vi "RSZVB Configure Power Bandwidth Average.vi"(5 "Meas Bandwidth (10.0e3)":dbl=10000.0 format="%^.3e", 6 "Average Factor (10)":i32=10, 7 "Average State (F: Off)":bool, 8 "error in (no error)":errorcluster {"code" format="%.0x"}, 9 "RF State (T: On)":bool=TRUE, 10 "Channel (1)":i32=1, 11 "VISA session":refnum<visa-resource-name>) -> (0 "error out":errorcluster {"code" format="%.0x"}, 3 "dup VISA session":refnum<visa-resource-name>)   [LabVIEW 2011]
doc: "This VI configures the power bandwidth average.\n\nRemote-control command(s):\nDIAGnostic:SERVice:RFPower\n[SENSe<Ch>:]BANDwidth[:RESolution]\n[SENSe<Ch>:]AVERage[:STATe]\n[SENSe<Ch>:]AVERage:COUNt"
panel:
  # "On\nOff"
  # "On\nOff"
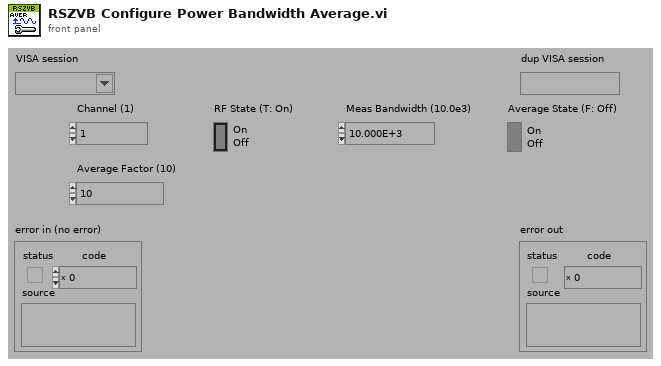
[diagram p1: front panel]
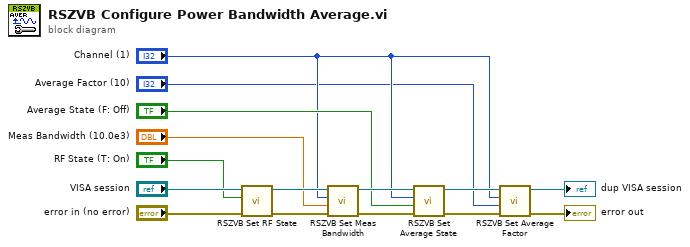
[diagram p0: block diagram]
diagram:
  n1 = call "RSZVB Set RF State.vi"("error in (no error)"="error in (no error)", "RF State (T: On)"="RF State (T: On)", "VISA session"="VISA session") -> ("error out"=w10:errorcluster, "dup VISA session"=w11:refnum<visa-resource-name>)  [unwired: 7 in]
  n2 = call "RSZVB Set Meas Bandwidth.vi"("error in (no error)"=w10, "Meas Bandwidth (10.0e3)"="Meas Bandwidth (10.0e3)", "Channel (1)"="Channel (1)", "VISA session"=w11) -> ("error out"=w9:errorcluster, "dup VISA session"=w8:refnum<visa-resource-name>)  [unwired: 6 in]
  n3 = call "RSZVB Set Average State.vi"("error in (no error)"=w9, "Average State (F: Off)"="Average State (F: Off)", "Channel (1)"="Channel (1)", "VISA session"=w8) -> ("error out"=w6:errorcluster, "dup VISA session"=w7:refnum<visa-resource-name>)  [unwired: 6 in]
  n4 = call "RSZVB Set Average Factor.vi"("error in (no error)"=w6, "Average Factor (10)"="Average Factor (10)", "Channel (1)"="Channel (1)", "VISA session"=w7) -> ("error out"=→"error out":errorcluster, "dup VISA session"=→"dup VISA session":refnum<visa-resource-name>)  [unwired: 6 in]
